vi "RunPython.vi"(0 "PathToScript":path, 1 "PathToUserDir":path, 2 "ScriptDir":string, 4 "keep cmd window open (f)":bool) -> (8 "standard output":string, 10 "error out":errorcluster)   [LabVIEW 2014, in "LV-PY.lvlib"]
uses:
  LV-PY.lvlib
panel:
  out "concatenated string":string
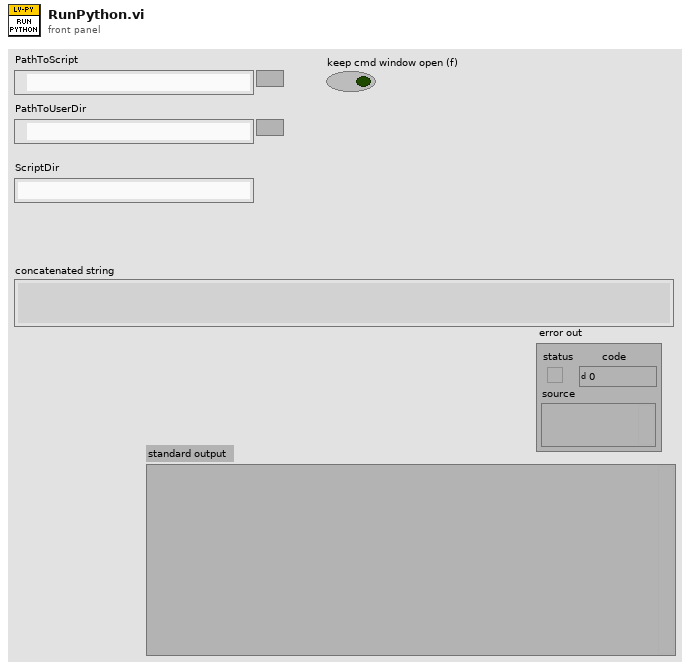
[diagram p1: front panel]
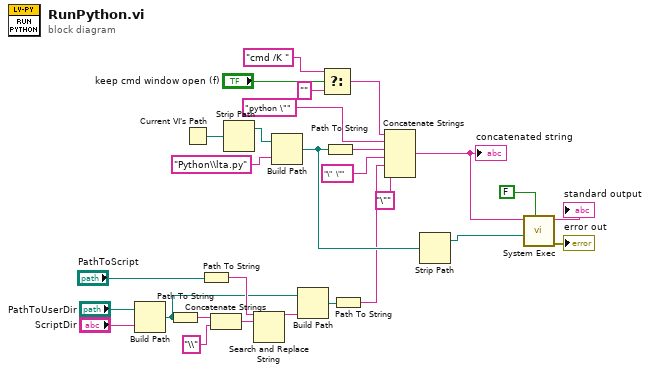
[diagram p0: block diagram]
diagram:
  n1 = Build Path(base path="PathToUserDir", name or relative path="ScriptDir") -> (appended path=w3:path)
  n2 = Path To String(path=w3) -> (string=w9:string)
  n3 = Current VI's Path() -> (path=w28:path)
  n4 = Path To String(path="PathToScript") -> (string=w7:string)
  n5 = Concatenate Strings(w9, "\\" ("string")) -> (w8:string)
  n6 = Strip Path(path=w28) -> (stripped path=w22:path)  [unwired: 1 out]
  n7 = Search and Replace String(input string=w7, search string=w8) -> (result string=w6:string)  [unwired: 6 in, 3 out]
  n8 = Build Path(base path=w22, name or relative path="Python\\lta.py") -> (appended path=w20:path)
  n9 = Build Path(base path=w3, name or relative path=w6) -> (appended path=w5:path)
  n10 = Select(t="cmd /K " ("string"), s="keep cmd window open (f)", f="") -> (s? t:f=w13:string)
  n11 = Path To String(path=w20) -> (string=w26:string)
  n12 = Path To String(path=w5) -> (string=w4:string)
  n13 = Concatenate Strings(w13, "python \"" ("command line"), w26, "\"  \"" ("string"), w4, "\"" ("string")) -> (w21:string)
  "concatenated string" <- w21
  n14 = Strip Path(path=w20) -> (stripped path=w19:path)  [unwired: 1 out]
  n15 = call <vilib>:"System Exec.vi"("wait until completion? (T)"=FALSE, "working directory"=w19, "command line"=w21) -> ("error out"=→"error out":errorcluster, "standard output"=→"standard output":string)  [unwired: 5 in, 2 out]
